vi "Hardware-DiffIOResultsCalPoints.vi"(10 "Diff IO Results":T2 {"Duty Cycle [%]" format="%#_3g"; "Frequency [Hz]" format="%#_3p"}, 11 "DIFF I/O State":T1) -> (3 "DiffIO State":bool[](array[boolean]))   [LabVIEW 2016, in "DSI-RT.lvlib"]
uses:
  DSI-RT.lvlib
  Shared/Typedefs/DiffIO-Results-Array.ctl
  <vilib>/Powertrain Controls/Device Drivers/DCM/Diff IO/RT/Results.ctl
  <vilib>/Powertrain Controls/Device Drivers/DCM/Tools/FPGA/8 Channels.ctl
  <vilib>/addons/Software Calibration Management/xSCM/CalPoint.xnode
  <vilib>/addons/Software Calibration Management/xSCM/ni_scm.dll
  <vilib>/Powertrain Controls/Device Drivers/DCM/Diff IO/RT/DCM - RT - Diff IO.lvlib
  <vilib>/Powertrain Controls/Device Drivers/DCM/Tools/FPGA/DCM - FPGA - Tools.lvlib
  Shared/DSI-Shared.lvlib
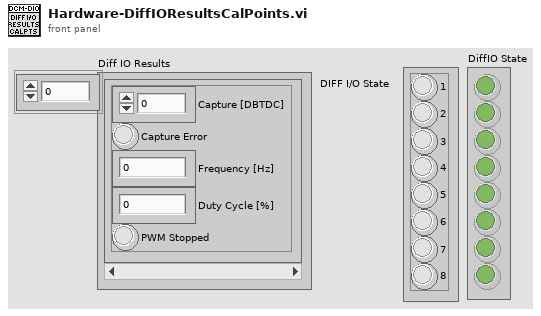
[diagram p1: front panel]
types:
  T1 = typedef "DCM - FPGA - Tools.lvlib/8 Channels.ctl" = cluster{"1":bool, "2":bool, "3":bool, "4":bool, "5":bool, "6":bool, "7":bool, "8":bool}
  T2 = typedef "DSI-Shared.lvlib/DiffIO-Results-Array.ctl" = T3[]
  T3 = typedef "DCM - RT - Diff IO.lvlib/Results.ctl" = cluster{"Capture [DBTDC]":sgl, "Capture Error":bool, "Frequency [Hz]":sgl, "Duty Cycle [%]":sgl, "PWM Stopped":bool}
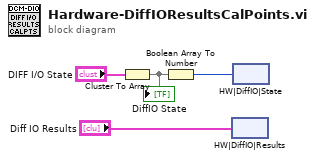
[diagram p0: block diagram]
diagram:
  n1 = Cluster To Array(cluster="DIFF I/O State") -> (array=w3:bool[])
  "DiffIO State" <- w3
  n2 = Boolean Array To Number(Boolean array=w3) -> (number=w2:u32)
  n3 = xnode "HW|DiffIO|Results"("Value"="Diff IO Results") -> ()
  n4 = xnode "HW|DiffIO|State"("Value"=w2) -> ()
